vi "Set Network Config.vi"(8 "error in (no error)":errorcluster, 10 "Network Config":T2={"Use DHCP"=FALSE, "IP settings"={"IP address"="0.0.0.0", "DNS name"="", "subnet mask"="0.0.0.0", "gateway"="0.0.0.0", "DNS server"="0.0.0.0"}}, 11 "MAC Address":string="\u0000\u0000\u0000\u0000\u0000\u0000") -> (0 "error out":errorcluster, 2 "IP settings after restart":T1)   [LabVIEW 2011]
doc: "Sets network configuration of a remote RT system.\n\n\nVersion 1.0 - 02/13/2013\n\nPhaeron, Inc.\nwww.phaeron.com\ninfo@phaeron.com"
uses:
  <vilib>/real-time/NI_Real-Time Libraries.lvlib
  <vilib>/real-time/rtutility.llb/RT Apply Target Network Settings (DHCP).vi
  <vilib>/real-time/rtutility.llb/RT Apply Target Network Settings (Static).vi
  Network Config.ctl
  <vilib>/real-time/rtutility.llb/subVIs/IP Settings.ctl
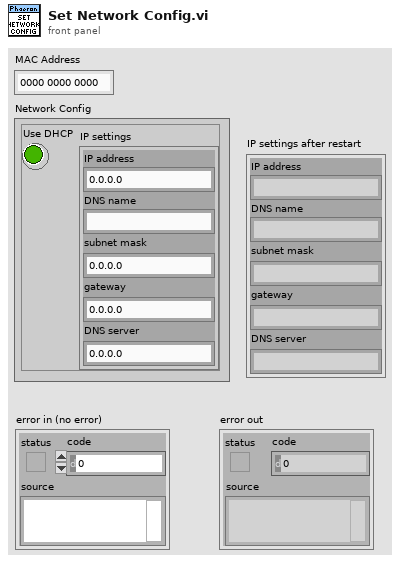
[diagram p1: front panel]
types:
  T1 = typedef "NI_Real-Time Libraries.lvlib/IP Settings.ctl" = cluster{"IP address":string, "DNS name":string, "subnet mask":string, "gateway":string, "DNS server":string}
  T2 = typedef "Network Config.ctl" = cluster{"Use DHCP":bool, "IP settings":T1}
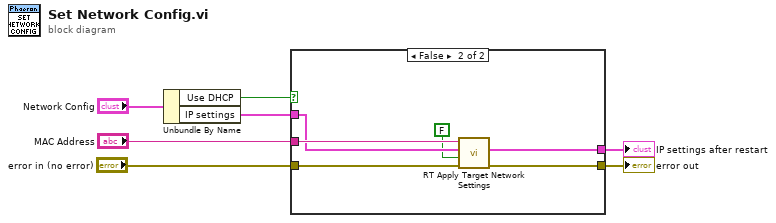
[diagram p0: block diagram]
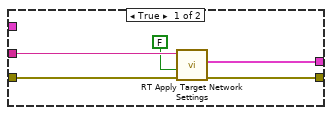
[diagram p2: hidden frame]
diagram:
  n1 = Unbundle By Name("Network Config") -> ("Use DHCP"=w5:bool, "IP settings"=w2:T1)
  n2 = case shown="False" w5 {
    tunnel: "MAC Address" -> [w12 w18]
    tunnel: "error in (no error)" -> [w11 w17]
    tunnel: [w10 w16] -> w3
    tunnel: w2 -> [_ w15]
    tunnel: [w8 w13] -> w1
    frame True {
      n3 = call-poly <vilib>:"RT Apply Target Network Settings.vi"("error in (no error)"=w11, "halt if TCP/IP fails? (T)"=FALSE, "MAC address"=w12) -> ("error out"=w10:errorcluster, "IP settings after restart"=w8:T1)  [unwired: 6 in, 1 out]
    }
    frame False {
      n4 = call-poly <vilib>:"RT Apply Target Network Settings.vi"("error in (no error)"=w17, "halt if TCP/IP fails? (T)"=FALSE, "IP settings"=w15, "MAC address"=w18) -> ("error out"=w16:errorcluster, "IP settings after restart"=w13:T1)  [unwired: 5 in, 1 out]
    }
  }
  "error out" <- w3
  "IP settings after restart" <- w1
